vi "Get Output FIFOs.vi"(11 "Output Process in":refnum<class "Random Process.lvclass">) -> (2 "Output FIFOs":refnum<k33>, 3 "Output Process out":refnum<class "Random Process.lvclass">)   [LabVIEW 2019, in "TimingDRV Engine.lvlib" / "Random Process.lvclass"]
uses:
  Random Process.lvclass
  Random Process.lvclass/Random Process.ctl
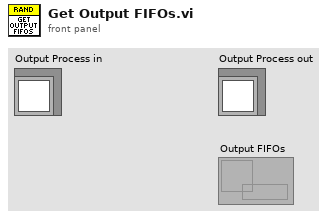
[diagram p1: front panel]
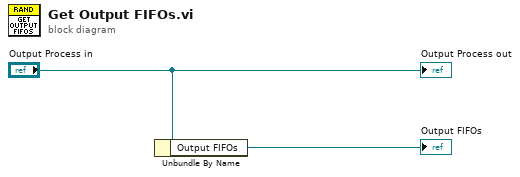
[diagram p0: block diagram]
diagram:
  n1 = Unbundle By Name("Output Process in") -> ("Output FIFOs"=→"Output FIFOs":refnum<k33>)
  "Output Process out" <- "Output Process in"
